vi "TopLevel.vi"() -> ()   [LabVIEW 2011]
uses:
  Globals.vi
panel:
  out "YPos 2":i32
  out "XPos 2":i32
  out "?":string
  in  "PC connection port":u16(ring) items=["PCI board", "COM 1", "TPL1", "COM3"]
  in  "Zabs":dbl
  in  "SetZspeed":bool
  in  "Zspeed":dbl=250.0
  out "ZPos":i32
  out "ZMoved":bool
  in  "Location":dbl
  in  "ZMoveAbs":bool
  in  "ZDown":bool
  in  "ZUp":bool
  in  "ScanStop":bool
  in  "ResetXY":bool
  in  "SetXY":bool
  in  "XYSpeed":dbl=11999.99824166298
  out "ShutterMoved":bool
  in  "Shutter Control":bool
  out "Temperature":sgl
  out "Position":i16
  out "WheelMoved":bool
  in  "MoveAbs":bool
  in  "YAbs":dbl
  in  "XAbs":dbl
  out "Shutter_3":bool
  out "Shutter_2":bool
  out "Shutter_1":bool
  out "StageMoved":bool
  in  "Previous":bool
  in  "Home":bool
  in  "Next":bool
  in  "Back":bool
  in  "Forward":bool
  in  "Right":bool
  in  "Left":bool
  in  "stop":bool
  in  "Stage Move":bool
  in  "YMove":dbl=1000.0
  in  "XMove":dbl=1000.0
  # "Prior DLL LabView Demonstration with Active X"
  # "IScan Methods"
  # "IFilter Methods"
  # "Z Axis Control"
  # "IStage Methods"
  # "Absolute Location"
  # "Z Axis Speed"
  # "Reset XY Defaults"
  # "Stage Location"
  # "Move Absolute"
  # "Shutter Sensors"
  # "Stop all motion"
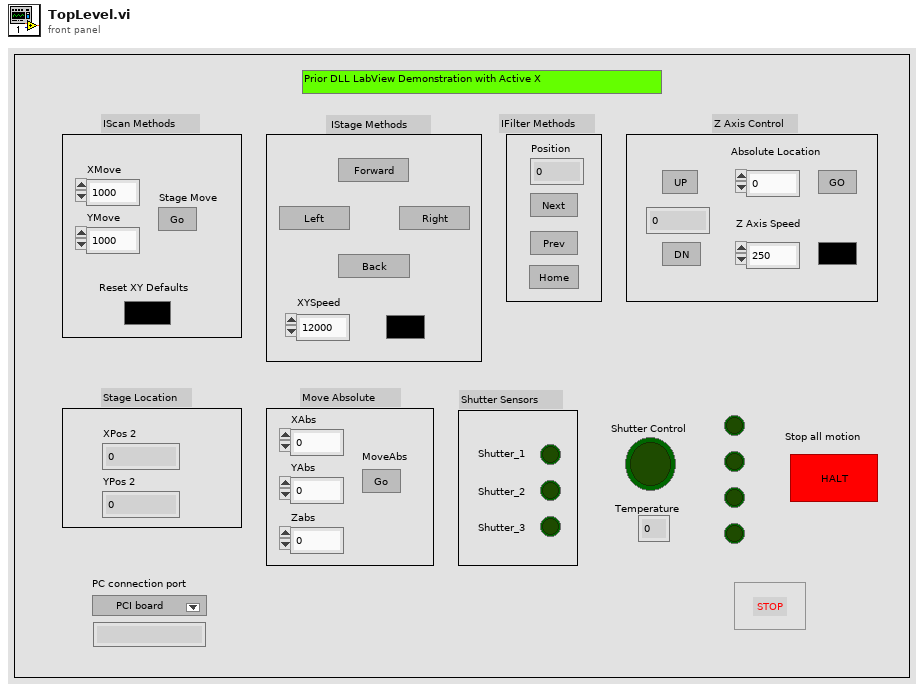
[diagram p1: front panel]
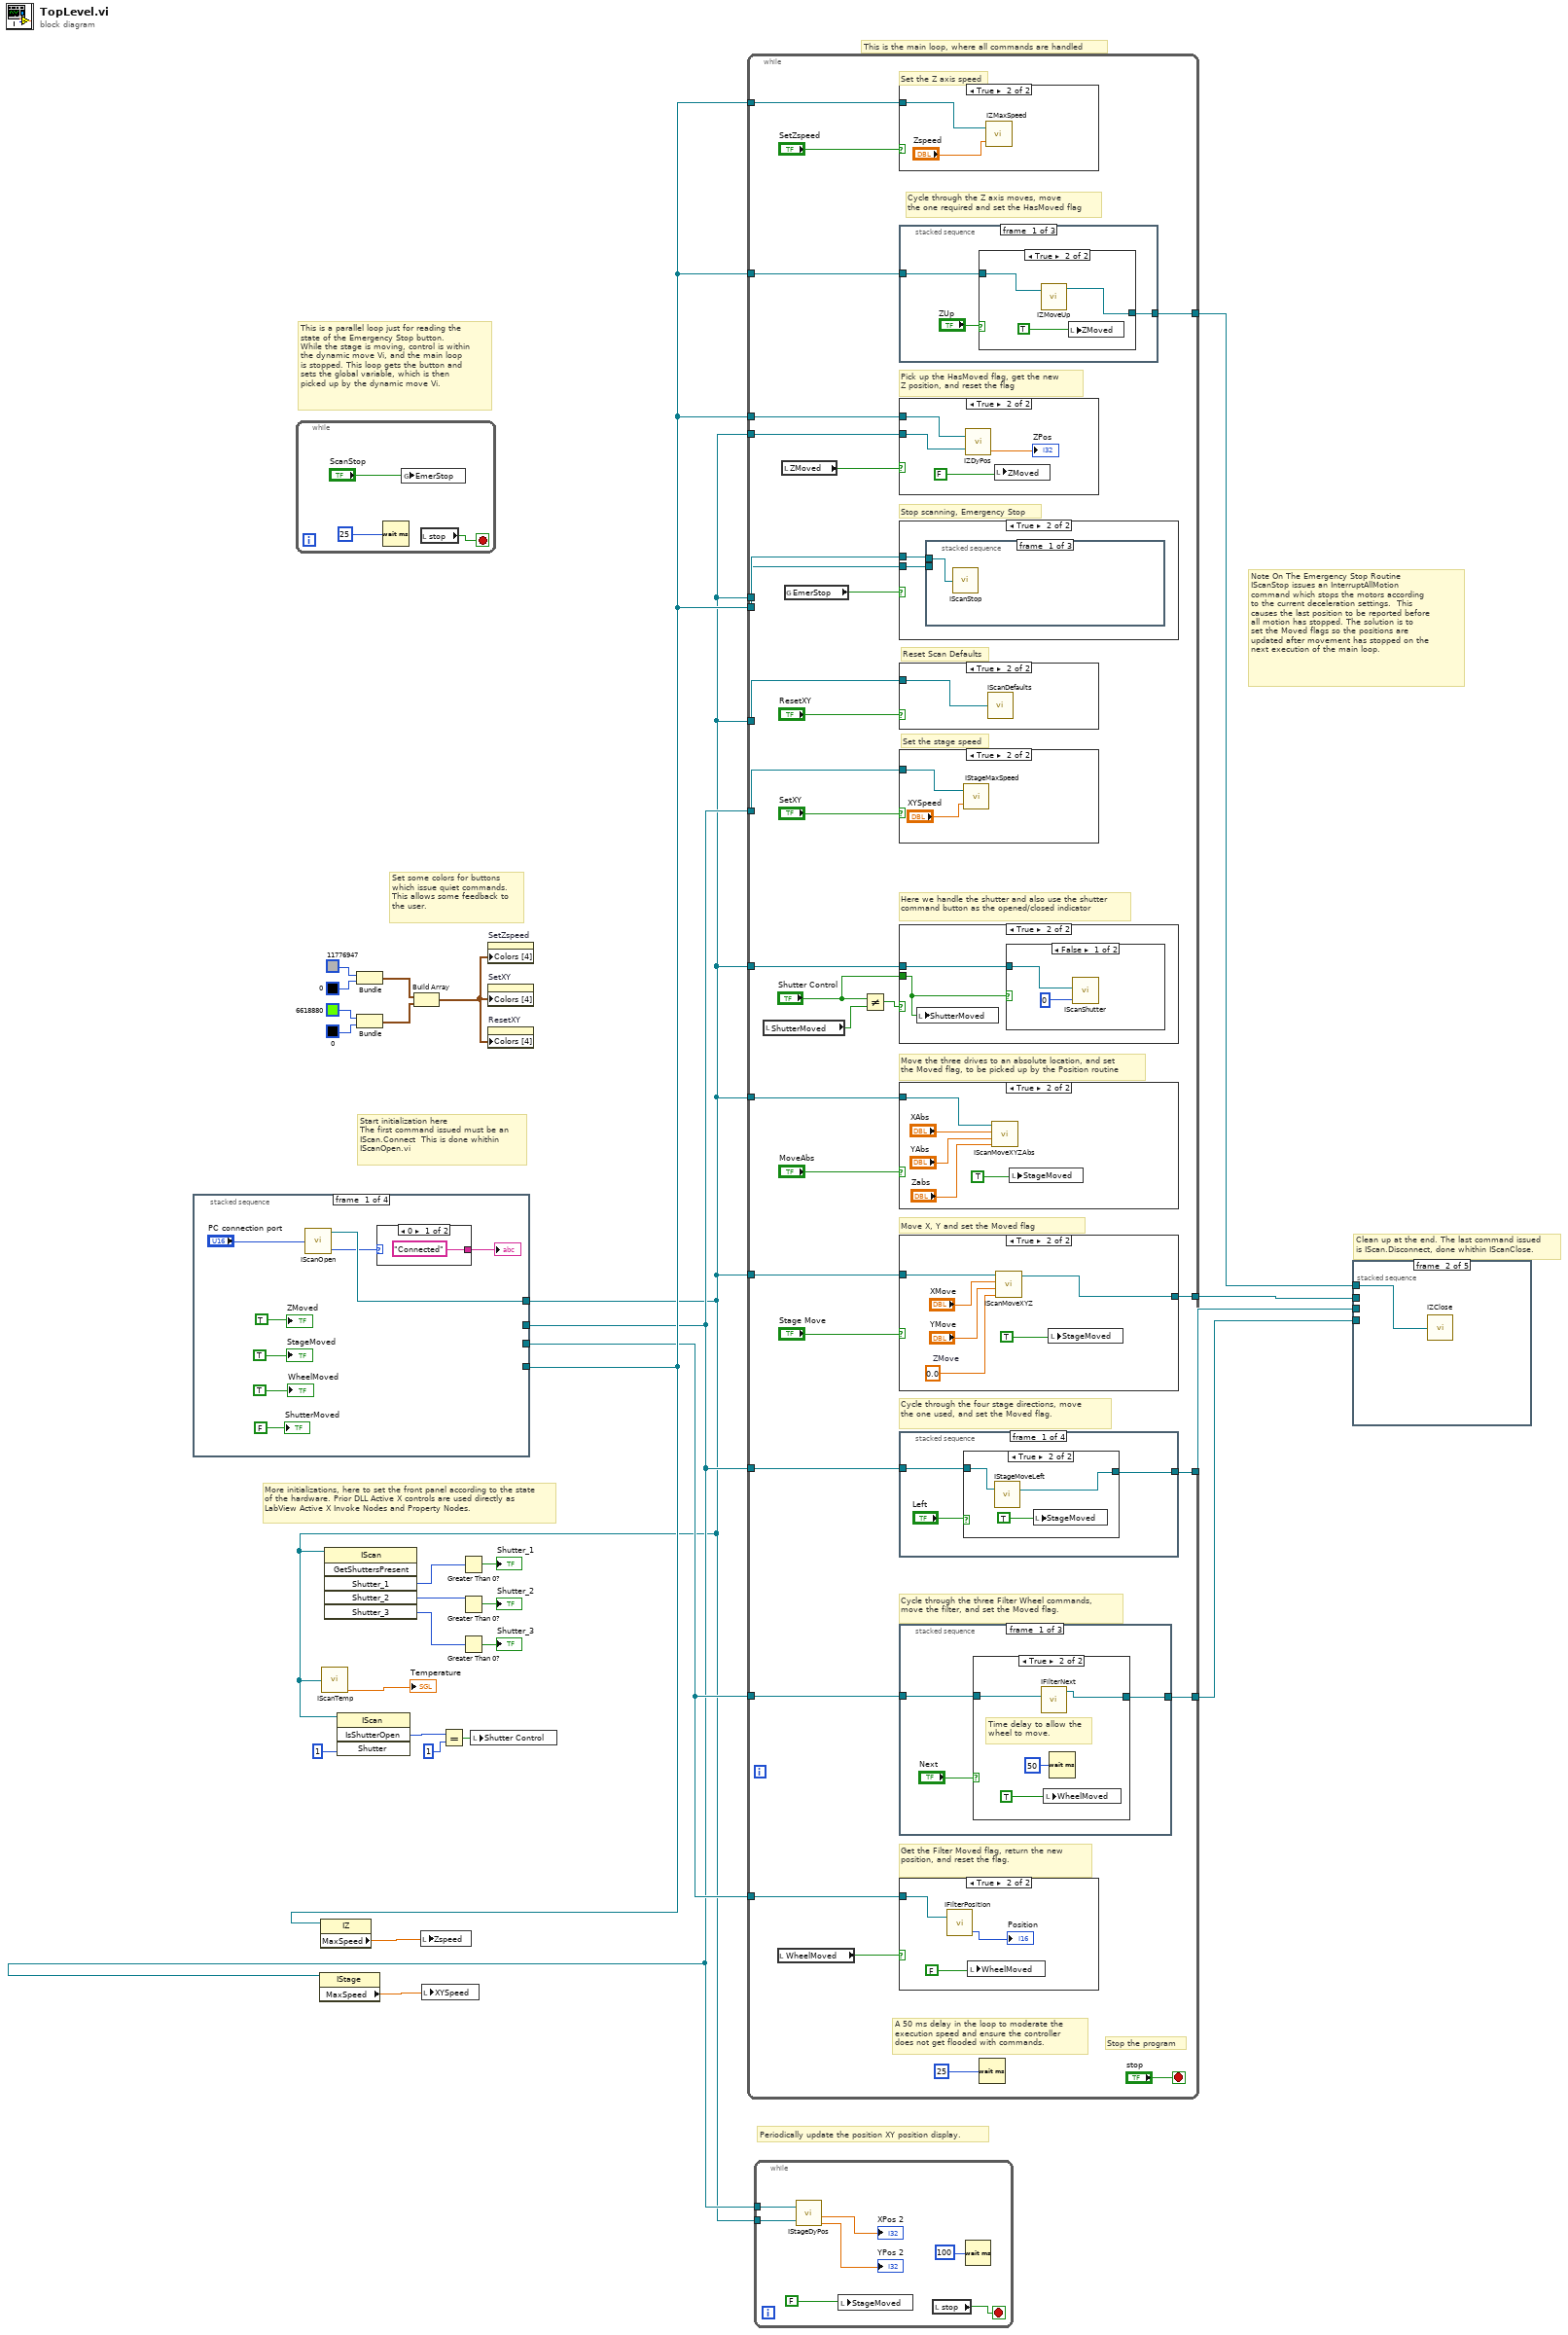
[diagram p0: block diagram]
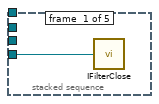
[diagram p2: hidden frame]
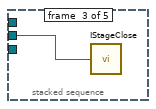
[diagram p3: hidden frame]
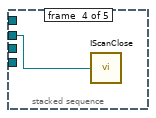
[diagram p4: hidden frame]
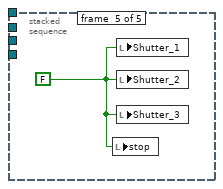
[diagram p5: hidden frame]
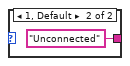
[diagram p6: hidden frame]
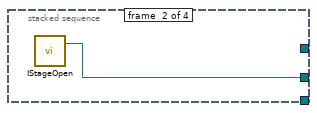
[diagram p7: hidden frame]
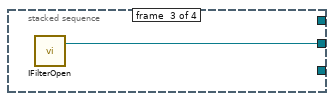
[diagram p8: hidden frame]
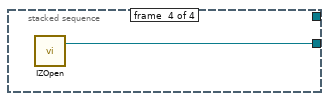
[diagram p9: hidden frame]
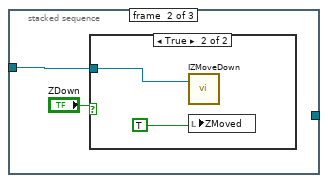
[diagram p13: hidden frame]
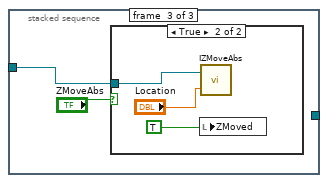
[diagram p15: hidden frame]
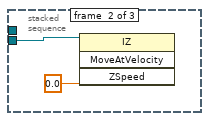
[diagram p18: hidden frame]
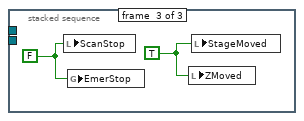
[diagram p19: hidden frame]
diagram:
  # "Periodically update the position XY position display."
  # "Note On The Emergency Stop Routine\nIScanStop issues an InterruptAllMotion\ncommand which stops the motors according\nto the current deceleration settings.  This\ncauses the last position to be reported before\nall motion has stopped. The solution is to\nset the Moved flags so the positions are\nupdated after movement has stopped on the\nnext execution of the main loop."
  # "This is a parallel loop just for reading the\nstate of the Emergency Stop button.\nWhile the stage is moving, control is within\nthe dynamic move Vi, and the main loop\nis stopped. This loop gets the button and\nsets the global variable, which is then\npicked up by the dynamic move Vi."
  # "This is the main loop, where all commands are handled"
  # "Clean up at the end. The last command issued\nis IScan.Disconnect, done whithin IScanClose."
  # "More initializations, here to set the front panel according to the state of the hardware. Prior DLL Active X controls are used directly as LabView Active X Invoke Nodes and Property Nodes."
  # "Start initialization here\nThe first command issued must be an\nIScan.Connect  This is done whithin\nIScanOpen.vi"
  # "Set some colors for buttons\nwhich issue quiet commands.\nThis allows some feedback to\nthe user."
  n1 = stacked-sequence {
    tunnel: [w33 _ _ _] -> w1
    tunnel: [_ w39 _ _] -> w2
    tunnel: [_ _ w40 _] -> w3
    tunnel: [_ _ _ w41] -> w4
    frame #0 {
      n2 = call "IScanOpen.vi"("Port"="PC connection port") -> ("PRIORLib.IScanOut"=w33:refnum<k7>, "Return"=w30:i32)  [unwired: 1 out]
      n3 = case shown="0" w30 {
        tunnel: ["Connected" "Unconnected"] -> w29
        frame 0 {
        }
        frame 1, Default {
        }
      }
      "?" <- w29
      "StageMoved" <- TRUE
      "WheelMoved" <- TRUE
      "ShutterMoved" <- FALSE
      "ZMoved" <- TRUE
    }
    frame #1 {
      n4 = call "IStageOpen.vi"() -> ("PRIORLib.IStageOut"=w39:refnum<k7>)  [unwired: 1 in, 1 out]
    }
    frame #2 {
      n5 = call "IFilterOpen.vi"() -> ("PRIORLib.IFilterOut"=w40:refnum<k7>)  [unwired: 1 in, 1 out]
    }
    frame #3 {
      n6 = call "IZOpen.vi"() -> ("PRIORLib.IZOut"=w41:refnum<k7>)  [unwired: 1 in, 1 out]
    }
  }
  n7 = while {
    stop <- w42 stop-if-true
    n8 = Wait (ms)(milliseconds to wait=u32 25) -> ()  [unwired: 1 out]
    n9 = global write "Globals.vi" "EmerStop"("ScanStop") -> ()
    n10 = local read "stop"() -> (w42:bool)
  }
  n11 = property class="IStage"(reference=w2) -> ("MaxSpeed"=w18:dbl)  [unwired: 1 in, 2 out]
  n12 = property class="IZ"(reference=w4) -> ("MaxSpeed"=w16:dbl)  [unwired: 1 in, 2 out]
  n13 = call "IScanTemp.vi"("PRIORLib.IScanIn"=w1) -> ("Temperature"=→"Temperature":sgl)  [unwired: 3 out]
  n14 = invoke class="IScan" method="GetShuttersPresent"(reference=w1) -> ("Shutter_1"=w21:i32, "Shutter_2"=w25:i32, "Shutter_3"=w23:i32)  [unwired: 5 in, 3 out]
  n15 = invoke on="Invoke Node" class="IScan" method="IsShutterOpen"(reference=w1, "Shutter"=1) -> ("IsShutterOpen"=w14:i32)  [unwired: 2 in, 3 out]
  n16 = Bundle(u32 11776947, u32 0) -> (w7:cluster{u32, u32})  [unwired: 1 in]
  n17 = Bundle(u32 6618880, u32 0) -> (w6:cluster{u32, u32})  [unwired: 1 in]
  n18 = Build Array(w7, w6) -> (w5:cluster{u32, u32}[])
  n19 = local write "Zspeed"(w16) -> ()
  n20 = local write "XYSpeed"(w18) -> ()
  n21 = Equal?(x=w14, y=1) -> (x = y?=w12:bool)
  n22 = Greater Than 0?(x=w21) -> (x > 0?=→"Shutter_1":bool)
  n23 = Greater Than 0?(x=w25) -> (x > 0?=→"Shutter_2":bool)
  n24 = Greater Than 0?(x=w23) -> (x > 0?=→"Shutter_3":bool)
  n25 = local write "Shutter Control"(w12) -> ()
  n26 = property on="SetZspeed" class="Bool"("Colors [4]"=w5) -> ()  [unwired: 2 in, 2 out]
  n27 = property on="SetXY" class="Bool"("Colors [4]"=w5) -> ()  [unwired: 2 in, 2 out]
  n28 = property on="ResetXY" class="Bool"("Colors [4]"=w5) -> ()  [unwired: 2 in, 2 out]
  n29 = while {
    tunnel: w1 -> [w75]
    tunnel: [w72] -> w28
    tunnel: w2 -> [w71]
    tunnel: [w70] -> w27
    tunnel: [w69] -> w26
    tunnel: w1 -> [w68]
    tunnel: w1 -> [w62]
    tunnel: w3 -> [w61]
    tunnel: w3 -> [w60]
    tunnel: w2 -> [w59]
    tunnel: w1 -> [w57]
    tunnel: w1 -> [w48]
    tunnel: w4 -> [w55]
    tunnel: [w54] -> w17
    tunnel: w4 -> [w53]
    tunnel: w1 -> [w52]
    tunnel: w4 -> [w49]
    tunnel: w4 -> [w45]
    stop <- "stop" stop-if-true
    # "A 50 ms delay in the loop to moderate the\nexecution speed and ensure the controller\ndoes not get flooded with commands."
    # "Stop the program"
    # "Get the Filter Moved flag, return the new position, and reset the flag."
    # "Cycle through the three Filter Wheel commands,\nmove the filter, and set the Moved flag."
    # "Cycle through the four stage directions, move\nthe one used, and set the Moved flag."
    # "Move X, Y and set the Moved flag"
    # "Move the three drives to an absolute location, and set\nthe Moved flag, to be picked up by the Position routine"
    # "Here we handle the shutter and also use the shutter\ncommand button as the opened/closed indicator"
    # "Set the stage speed"
    # "Reset Scan Defaults"
    # "Stop scanning, Emergency Stop"
    # "Pick up the HasMoved flag, get the new\nZ position, and reset the flag"
    # "Cycle through the Z axis moves, move\nthe one required and set the HasMoved flag"
    # "Set the Z axis speed"
    n30 = local read "ShutterMoved"() -> (w65:bool)
    n31 = local read "WheelMoved"() -> (w66:bool)
    n32 = local read "ZMoved"() -> (w51:bool)
    n33 = global read "Globals.vi" "EmerStop"() -> (w46:bool)
    n34 = Not Equal?(x="Shutter Control", y=w65) -> (x != y?=w64:bool)
    n35 = case shown="True" "SetZspeed" {
      tunnel: w49 -> [_ w77]
      frame False {
      }
      frame True {
        n36 = call "IZMaxSpeed.vi"("ZSpeed"="Zspeed", "PRIORLib.IZIn"=w77) -> ()  [unwired: 2 out]
      }
    }
    n37 = stacked-sequence {
      tunnel: w55 -> [w83 w89 w93]
      tunnel: [w82 _ _] -> w54
      frame #0 {
        n38 = case shown="True" "ZUp" {
          tunnel: w83 -> [w85 w87]
          tunnel: [w85 w86] -> w82
          frame False {
          }
          frame True {
            n39 = call "IZMoveUp.vi"("PRIORLib.IZIn"=w87) -> ("PRIORLib.IZOut"=w86:refnum<k7>)  [unwired: 1 in, 2 out]
            n40 = local write "ZMoved"(TRUE) -> ()
          }
        }
      }
      frame #1 {
        n41 = case shown="True" "ZDown" {
          tunnel: w89 -> [_ w91]
          frame False {
          }
          frame True {
            n42 = call "IZMoveDown.vi"("PRIORLib.IZIn"=w91) -> ()  [unwired: 1 in, 3 out]
            n43 = local write "ZMoved"(TRUE) -> ()
          }
        }
      }
      frame #2 {
        n44 = case shown="True" "ZMoveAbs" {
          tunnel: w93 -> [_ w96]
          frame False {
          }
          frame True {
            n45 = local write "ZMoved"(TRUE) -> ()
            n46 = call "IZMoveAbs.vi"("PRIORLib.IZIn"=w96, "Location"="Location") -> ()  [unwired: 3 out]
          }
        }
      }
    }
    n47 = case shown="True" w51 {
      tunnel: w53 -> [_ w79]
      tunnel: w52 -> [_ w78]
      frame False {
      }
      frame True {
        n48 = call "IZDyPos.vi"("PRIORLib.IZIn"=w79, "PRIORLib.IScanIn"=w78) -> ("ZPos"=→"ZPos":dbl)  [unwired: 2 out]
        n49 = local write "ZMoved"(FALSE) -> ()
      }
    }
    n50 = case shown="True" w46 {
      tunnel: w48 -> [_ w99]
      tunnel: w45 -> [_ w98]
      frame False {
      }
      frame True {
        n51 = stacked-sequence {
          tunnel: w99 -> [w100 _ _]
          tunnel: w98 -> [_ w102 _]
          frame #0 {
            n52 = call "IScanStop.vi"("PRIORLib.IScanIn"=w100) -> ()  [unwired: 3 out]
          }
          frame #1 {
            n53 = invoke class="IZ" method="MoveAtVelocity"(reference=w102, "ZSpeed"=0.0) -> ()  [unwired: 2 in, 4 out]
          }
          frame #2 {
            w103 = TRUE
            w104 = FALSE
            n54 = local write "ScanStop"(w104) -> ()
            n55 = global write "Globals.vi" "EmerStop"(w104) -> ()
            n56 = local write "ZMoved"(w103) -> ()
            n57 = local write "StageMoved"(w103) -> ()
          }
        }
      }
    }
    n58 = case shown="True" "ResetXY" {
      tunnel: w57 -> [_ w105]
      frame False {
      }
      frame True {
        n59 = call "IScanDefaults.vi"("PRIORLib.IScanIn"=w105) -> ()  [unwired: 3 out]
      }
    }
    n60 = case shown="True" "SetXY" {
      tunnel: w59 -> [_ w106]
      frame False {
      }
      frame True {
        n61 = call "IStageMaxSpeed.vi"("XYSpeed"="XYSpeed", "PRIORLib.IStageIn"=w106) -> ()  [unwired: 2 out]
      }
    }
    n62 = case shown="True" w64 {
      tunnel: "Shutter Control" -> [_ w109]
      tunnel: w62 -> [_ w108]
      frame False {
      }
      frame True {
        n63 = local write "ShutterMoved"(w109) -> ()
        n64 = case shown="False" w109 {
          tunnel: w108 -> [w111 w113]
          frame False {
            n65 = call "IScanShutter.vi"("OpenNotClose"=0, "PRIORLib.IScanIn"=w111) -> ()  [unwired: 1 in, 3 out]
          }
          frame True {
            n66 = call "IScanShutter.vi"("OpenNotClose"=1, "PRIORLib.IScanIn"=w113) -> ()  [unwired: 1 in, 3 out]
          }
        }
      }
    }
    n67 = case shown="True" "MoveAbs" {
      tunnel: w68 -> [_ w120]
      frame False {
      }
      frame True {
        n68 = call "IScanMoveXYZAbs.vi"("ZPos"="Zabs", "YPos"="YAbs", "XPos"="XAbs", "PRIORLib.IScanIn"=w120) -> ()  [unwired: 3 out]
        n69 = local write "StageMoved"(TRUE) -> ()
      }
    }
    n70 = case shown="True" "Stage Move" {
      tunnel: w75 -> [w169 w174]
      tunnel: [w169 w170] -> w72
      frame False {
      }
      frame True {
        w171 = 0.0  # ZMove
        n71 = call "IScanMoveXYZ.vi"("ZPos"=w171, "YPos"="YMove", "XPos"="XMove", "PRIORLib.IScanIn"=w174) -> ("PRIORLib.IScanOut"=w170:refnum<k7>)  [unwired: 2 out]
        n72 = local write "StageMoved"(TRUE) -> ()
      }
    }
    n73 = stacked-sequence {
      tunnel: w71 -> [w146 w152 w158 w164]
      tunnel: [w145 _ _ _] -> w70
      frame #0 {
        n74 = case shown="True" "Left" {
          tunnel: w146 -> [w147 w150]
          tunnel: [w147 w149] -> w145
          frame False {
          }
          frame True {
            n75 = call "IStageMoveLeft.vi"("PRIORLib.IStageIn"=w150) -> ("PRIORLib.IStageOut"=w149:refnum<k7>)  [unwired: 1 in, 2 out]
            n76 = local write "StageMoved"(TRUE) -> ()
          }
        }
      }
      frame #1 {
        n77 = case shown="True" "Right" {
          tunnel: w152 -> [w153 w156]
          tunnel: [w153 w155] -> _
          frame False {
          }
          frame True {
            n78 = call "IStageMoveRight.vi"("PRIORLib.IStageIn"=w156) -> ("PRIORLib.IStageOut"=w155:refnum<k7>)  [unwired: 1 in, 2 out]
            n79 = local write "StageMoved"(TRUE) -> ()
          }
        }
      }
      frame #2 {
        n80 = case shown="True" "Back" {
          tunnel: w158 -> [w159 w160]
          tunnel: [w159 w161] -> _
          frame False {
          }
          frame True {
            n81 = call "IStageMoveBack.vi"("PRIORLib.IStageIn"=w160) -> ("PRIORLib.IStageOut"=w161:refnum<k7>)  [unwired: 1 in, 2 out]
            n82 = local write "StageMoved"(TRUE) -> ()
          }
        }
      }
      frame #3 {
        n83 = case shown="True" "Forward" {
          tunnel: w164 -> [w165 w166]
          tunnel: [w165 w167] -> _
          frame False {
          }
          frame True {
            n84 = call "IStageMoveForward.vi"("PRIORLib.IStageIn"=w166) -> ("PRIORLib.IStageOut"=w167:refnum<k7>)  [unwired: 1 in, 2 out]
            n85 = local write "StageMoved"(TRUE) -> ()
          }
        }
      }
    }
    n86 = stacked-sequence {
      tunnel: [w123 _ _] -> w69
      tunnel: w61 -> [w122 w130 w137]
      frame #0 {
        n87 = case shown="True" "Next" {
          tunnel: [w125 w126] -> w123
          tunnel: w122 -> [w125 w127]
          frame False {
          }
          frame True {
            # "Time delay to allow the\nwheel to move."
            n88 = call "IFilterNext.vi"("PRIORLib.IFilterIn"=w127) -> ("PRIORLib.IFilterrOut"=w126:refnum<k7>)  [unwired: 1 in, 2 out]
            n89 = local write "WheelMoved"(TRUE) -> ()
            n90 = Wait (ms)(milliseconds to wait=u32 50) -> ()  [unwired: 1 out]
          }
        }
      }
      frame #1 {
        n91 = case shown="True" "Previous" {
          tunnel: [w132 w134] -> _
          tunnel: w130 -> [w132 w133]
          frame False {
          }
          frame True {
            n92 = call "IFilterPrevious.vi"("PRIORLib.IFilterIn"=w133) -> ("PRIORLib.IFilterrOut"=w134:refnum<k7>)  [unwired: 1 in, 2 out]
            n93 = local write "WheelMoved"(TRUE) -> ()
            n94 = Wait (ms)(milliseconds to wait=u32 50) -> ()  [unwired: 1 out]
          }
        }
      }
      frame #2 {
        n95 = case shown="True" "Home" {
          tunnel: [w139 w142] -> _
          tunnel: w137 -> [w139 w140]
          frame False {
          }
          frame True {
            n96 = local write "WheelMoved"(TRUE) -> ()
            n97 = call "IFilterHome.vi"("PRIORLib.IFilterIn"=w140) -> ("PRIORLib.IFilterrOut"=w142:refnum<k7>)  [unwired: 1 in, 2 out]
            n98 = Wait (ms)(milliseconds to wait=u32 500) -> ()  [unwired: 1 out]
          }
        }
      }
    }
    n99 = case shown="True" w66 {
      tunnel: w60 -> [_ w114]
      frame False {
      }
      frame True {
        n100 = call "IFilterPosition.vi"("PRIORLib.IFilterIn"=w114) -> ("Position"=→"Position":i16)  [unwired: 1 in, 2 out]
        n101 = local write "WheelMoved"(FALSE) -> ()
      }
    }
    n102 = Wait (ms)(milliseconds to wait=u32 25) -> ()  [unwired: 1 out]
  }
  n103 = while {
    tunnel: w2 -> [w177]
    tunnel: w1 -> [w176]
    stop <- w178 stop-if-true
    n104 = call "IStageDyPos.vi"("PRIORLib.IStageIn"=w177, "PRIORLib.IScanIn"=w176) -> ("XPos"=→"XPos 2":dbl, "YPos"=→"YPos 2":dbl)  [unwired: 2 out]
    n105 = local write "StageMoved"(FALSE) -> ()
    n106 = local read "stop"() -> (w178:bool)
    n107 = Wait (ms)(milliseconds to wait=100) -> ()  [unwired: 1 out]
  }
  n108 = stacked-sequence {
    tunnel: w28 -> [_ _ _ w186 _]
    tunnel: w27 -> [_ _ w185 _ _]
    tunnel: w26 -> [w183 _ _ _ _]
    tunnel: w17 -> [_ w184 _ _ _]
    frame #0 {
      n109 = call "IFilterClose.vi"("PRIORLib.IFilter"=w183) -> ()  [unwired: 1 out]
    }
    frame #1 {
      n110 = call "IZClose.vi"("PRIORLib.IZ"=w184) -> ()  [unwired: 1 out]
    }
    frame #2 {
      n111 = call "IStageClose.vi"("PRIORLib.IStage"=w185) -> ()  [unwired: 1 out]
    }
    frame #3 {
      n112 = call "IScanClose.vi"("PRIORLib.IScan"=w186) -> ()  [unwired: 2 out]
    }
    frame #4 {
      w187 = FALSE
      n113 = local write "stop"(w187) -> ()
      n114 = local write "Shutter_1"(w187) -> ()
      n115 = local write "Shutter_2"(w187) -> ()
      n116 = local write "Shutter_3"(w187) -> ()
    }
  }
